vi "Chat Message Callback.vi"(7 "Owner":refnum<class>, 11 "Message":refnum<class "Message.lvclass">) -> (0 "error out":errorcluster)   [LabVIEW 2020, in "LV Chat Client.lvclass"]
uses:
  LV Chat Client.lvclass
  <vilib>/IlluminatedG/lv-msg-simple/Stream-Simple-Msg/Message/Message.lvclass
  Data Types/Message.ctl
  3bb6c120-6c39-4e60-a368-f8a06dca41d0.vi
  3bb6c120-6c39-4e60-a368-f8a06dca41d0.vi/91ba9c5b-4e27-4c7a-b10f-814da5a466e2.vi
  <vilib>/IlluminatedG/lv-msg-simple/Stream-Simple-Msg/Message/Data and Type.vi
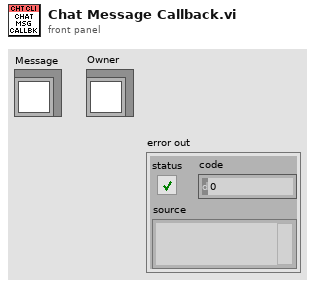
[diagram p1: front panel]
types:
  T1 = typedef "Message.ctl" = cluster{"From":string, "Time":dbl, "Message":string}
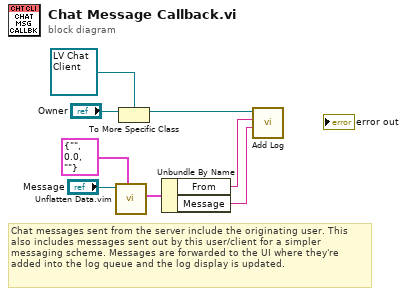
[diagram p0: block diagram]
diagram:
  # "Chat messages sent from the server include the originating user. This also includes messages sent out by this user/client for a simpler messaging scheme. Messages are forwarded to the UI where they're added into the log queue and the log display is updated."
  n1 = call "Unflatten Data.vim"("Data Type (String)"=T1 {"From"="", "Time"=0.0, "Message"=""} ("Message"), "Message in"="Message") -> ("Unflattened Data"=w6:T1)  [unwired: 7 in, 2 out]
  n2 = To More Specific Class(target class=refnum<class "LV Chat Client.lvclass"> refnum ("LV Chat Client.lvclass"), reference="Owner") -> (specific class reference=w3:refnum<class "LV Chat Client.lvclass">)  [unwired: 1 in, 1 out]
  n3 = Unbundle By Name(w6) -> ("From"=w2:string, "Message"=w1:string)
  n4 = call "Add Log.vi"("Message"=w1, "From (Client)"=w2, "LV Chat Client in"=w3) -> ()  [unwired: 7 in, 2 out]
